vi "Image_Handler.vi"(0 "Camera":T5, 5 "Data":T2={"system"={"info"={"menuSelect"=0, "version"=0, "serial"="Test Sample", "captureActive"=FALSE, "captureBegin"=FALSE, "emptyAndRefill"=FALSE}, "userInfo"={"operatorName"="", "date"=timestamp(2713993200 s since 1904-01-01)}, "camera"={"exposureTime"=0, "aperture"=enum."Item 0", "framerate"=0, "framerateMax"=500, "legacyAttributes"=FALSE}}, "connections"={"arduino"={"connection"="MRJ", "status"=FALSE, "openState"=FALSE, "emptyStart"=0}, "pump"={"connection"="MRJ", "status"=FALSE, "command"="", "dispenseSpeed"=100, "flushSize"=100}, "camera"={"cam1"={"connection"="", "status"=FALSE}, "cam2"={"connection"="", "status"=FALSE}}}, "queue"={"process"={"cam1"=refnum, "cam2"=refnum, "queueSize"=0}, "save"={"cam1"=refnum, "cam2"=refnum, "queueSize"=0}, "overloadThreshold"=0}, "imageProcess"={"cam1"={"preAllocation"={"image"="Station", "originalDisplay"="Station", "originalRgb"="Station", "binary"="Station", "save"="Station", "calibrationFull"=refnum, "calibrationDetect"=refnum}, "calibration"={"pathFull"=path "C:/Users/au540322/Desktop/IHS_Project/images/Debris/Debris_0/Debris_0_2019_06_01-23-32-49-686.PNG", "pathDetect"=path "C:/Users/au540322/Desktop/IHS_Project/images/Debris/Debris_0/Debris_0_2019_06_01-23-32-49-686.PNG", "ROI"={"Left"=0, "Top"=0, "Right"=0, "Bottom"=0, "Rotation"=0.0}}}, "cam2"={"preAllocation"={"image"=refnum, "originalDisplay"=refnum, "originalRgb"=refnum, "binary"=refnum, "save"=refnum, "calibrationFull"=refnum, "calibrationDetect"=refnum}, "calibration"={"pathFull"=path "C:/Users/au540322/Desktop/IHS_Project/images/Debris/Debris_0/Debris_0_2019_06_01-23-32-49-686.PNG", "pathDetect"=path "C:/Users/au540322/Desktop/IHS_Project/images/Debris/Debris_0/Debris_0_2019_06_01-23-32-49-686.PNG", "ROI"={"Left"=0, "Top"=0, "Right"=0, "Bottom"=0, "Rotation"=0.0}}}, "process"={"planeExtract"=refnum, "planeSubtract"=refnum, "cropMask"=refnum}, "detection"={"sampleTimeout"=500, "sizeThreshold"=500, "detectionRegionPct"=0.0}}, "sampleData"={"sampleId"="", "projectId"="", "voucherID"="", "speciesName"="", "collectionDate"=timestamp(2713993200 s since 1904-01-01), "sampleStation"="", "location"="", "lat"=0.0, "lon"=0.0, "determiner"="", "sex"="", "otherNotes"=""}, "Session In"=""} {"sampleData"."collectionDate" format="%<%Y-%m-%d>T"; "imageProcess"."detection"."sizeThreshold" min=1; "imageProcess"."cam2"."calibration"."ROI"."Rotation" format="%.2f"; "imageProcess"."cam2"."calibration"."ROI"."Left" scale=0.0..1024.0; "imageProcess"."cam2"."calibration"."ROI"."Right" scale=0.0..1024.0; "imageProcess"."cam1"."calibration"."ROI"."Rotation" format="%.2f"; "imageProcess"."cam1"."calibration"."ROI"."Left" scale=0.0..1024.0; "imageProcess"."cam1"."calibration"."ROI"."Right" scale=0.0..1024.0; "queue"."overloadThreshold" min=1; "queue"."save"."queueSize" min=1; "queue"."process"."queueSize" min=1; "connections"."pump"."flushSize" min=1; "connections"."pump"."dispenseSpeed" min=1; "system"."camera"."framerateMax" min=1; "system"."userInfo"."date" format="%<%Y-%m-%dT%H:%M:%S+%z>T"; "system"."info"."version" items=["Standard", "XL"]; "system"."info"."menuSelect" items=["Session Data", "Extended Setup", "Buffer", "Camera", "Dispenser", "Stats", "Connections"]}, 9 "Prev. sample":i32, 11 "Timeout in":i32) -> (2 "Detection error":errorcluster, 3 "Object":bool, 4 "Detected object":T1, 6 "Image Out":T1, 8 "Binary":T1, 10 "Sample nr":i32, 15 "Timeout out":i32)   [LabVIEW 2022 SP3]
uses:
  Camera_ID.ctl
  controls/Data.ctl
  <vilib>/userdefined/High Color/IMAQdx.ctl
  <vilib>/vision/Image Controls.llb/IMAQ Image.ctl
panel:
  out "error out 1":errorcluster
  out "error out 2":errorcluster
  in  "error in":errorcluster
  out "error out":errorcluster
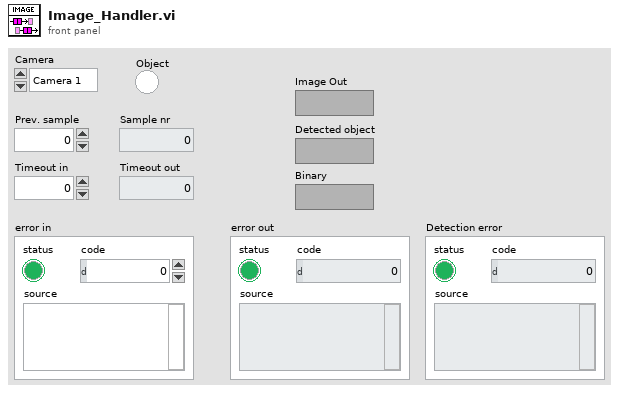
[diagram p1: front panel]
types:
  T1 = typedef "IMAQ Image.ctl" = refnum<image>
  T2 = typedef "Data.ctl" = cluster{"system":cluster{"info":cluster{"menuSelect":u16, "version":u16, "serial":string, "captureActive":bool, "captureBegin":bool, "emptyAndRefill":bool}, "userInfo":cluster{"operatorName":string, "date":timestamp}, "camera":cluster{"exposureTime":i32, "aperture":enum32{"Item 0", "Item 1", "Item 2", "Item 3"}, "framerate":i32, "framerateMax":i32, "legacyAttributes":bool}}, "connections":cluster{"arduino":cluster{"connection":refnum<visa-resource-name>, "status":bool, "openState":bool, "emptyStart":u32}, "pump":cluster{"connection":refnum<visa-resource-name>, "status":bool, "command":string, "dispenseSpeed":i32, "flushSize":i32}, "camera":cluster{"cam1":cluster{"connection":T3, "status":bool}, "cam2":cluster{"connection":T3, "status":bool}}}, "queue":cluster{"process":cluster{"cam1":refnum<queue>, "cam2":refnum<queue>, "queueSize":i32}, "save":cluster{"cam1":refnum<queue>, "cam2":refnum<queue>, "queueSize":i32}, "overloadThreshold":i32}, "imageProcess":cluster{"cam1":cluster{"preAllocation":cluster{"image":T1, "originalDisplay":T1, "originalRgb":T1, "binary":T1, "save":T1, "calibrationFull":T1, "calibrationDetect":T1}, "calibration":cluster{"pathFull":path, "pathDetect":path, "ROI":T4}}, "cam2":cluster{"preAllocation":cluster{"image":T1, "originalDisplay":T1, "originalRgb":T1, "binary":T1, "save":T1, "calibrationFull":T1, "calibrationDetect":T1}, "calibration":cluster{"pathFull":path, "pathDetect":path, "ROI":T4}}, "process":cluster{"planeExtract":T1, "planeSubtract":T1, "cropMask":T1}, "detection":cluster{"sampleTimeout":i32, "sizeThreshold":i32, "detectionRegionPct":dbl}}, "sampleData":cluster{"sampleId":string, "projectId":string, "voucherID":string, "speciesName":string, "collectionDate":timestamp, "sampleStation":string, "location":string, "lat":dbl, "lon":dbl, "determiner":string, "sex":string, "otherNotes":string}, "Session In":T3}
  T3 = typedef "IMAQdx.ctl" = refnum<k21>
  T4 = typedef "IMAQ Rectangle" = cluster{"Left":i32, "Top":i32, "Right":i32, "Bottom":i32, "Rotation":dbl}
  T5 = typedef "Camera_ID.ctl" = enum16{"Camera 1", "Camera 2"}
  T6 = cluster{"Image Pixels (U32)":u32[][], "Detect Movement":bool}
  T7 = cluster{"Global Rectangle":i32[], "Contours":cluster{"ID":enum32{"External", "Internal"}, "Type":u32, "Coordinates":i32[]}[]}
  T8 = cluster{"Timestamp":string, "Image Pixels (U32)":u32[][], "Prev. sample":i32, "Sample Data":dbl[], "ROI descriptor":cluster{"Global Rectangle":i32[], "Contours":cluster{"ID":enum32{"External", "Internal"}, "Type":u32, "Coordinates":i32[]}[]}}
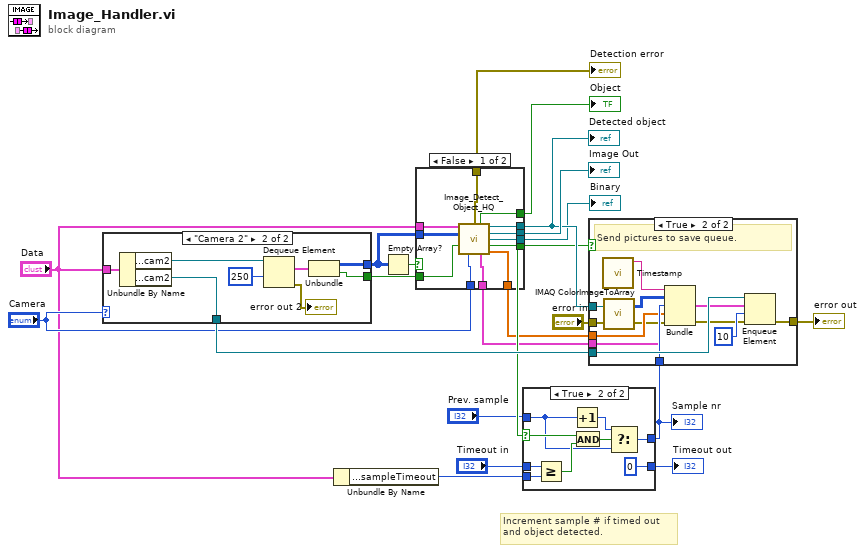
[diagram p0: block diagram]
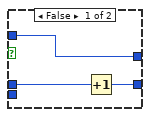
[diagram p2: hidden frame]
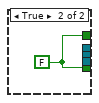
[diagram p4: hidden frame]
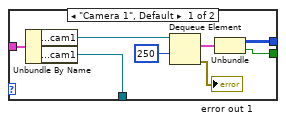
[diagram p5: hidden frame]
diagram:
  # "Increment sample # if timed out \nand object detected."
  n1 = case shown="\"Camera 2\"" "Camera" {
    tunnel: "Data" -> [w29 w37]
    tunnel: [w25 w32] -> w18
    tunnel: [w24 w31] -> w9
    tunnel: [w23 w30] -> w5
    frame "Camera 1", Default {
      n2 = Unbundle By Name(w29) -> ("queue.process.cam1"=w27:refnum<queue>, "queue.save.cam1"=w25:refnum<queue>)
      n3 = Dequeue Element(queue=w27, timeout in ms (-1)=250) -> (element=w22:T6, error out=→"error out 1":errorcluster)  [unwired: 1 in, 2 out]
      n4 = Unbundle(w22) -> ("Image Pixels (U32)"=w24:u32[][], "Detect Movement"=w23:bool)
    }
    frame "Camera 2" {
      n5 = Unbundle By Name(w37) -> ("queue.process.cam2"=w35:refnum<queue>, "queue.save.cam2"=w32:refnum<queue>)
      n6 = Dequeue Element(queue=w35, timeout in ms (-1)=250) -> (element=w34:T6, error out=→"error out 2":errorcluster)  [unwired: 1 in, 2 out]
      n7 = Unbundle(w34) -> ("Image Pixels (U32)"=w31:u32[][], "Detect Movement"=w30:bool)
    }
  }
  n8 = Unbundle By Name("Data") -> ("imageProcess.detection.sampleTimeout"=w11:i32)
  n9 = Empty Array?(array=w9) -> (empty?=w21:bool)
  n10 = case shown="False" w21 {
    tunnel: [w49 _] -> w19
    tunnel: [w41 w50] -> w14
    tunnel: "Data" -> [w48 _]
    tunnel: "Camera" -> [w47 _]
    tunnel: [w46 _] -> w20
    tunnel: w9 -> [w45 _]
    tunnel: [w44 w50] -> w6
    tunnel: w5 -> [w43 _]
    tunnel: [w42 _] -> w4
    tunnel: [w40 _] -> w3
    tunnel: [w39 _] -> w2
    tunnel: [w38 _] -> w1
    frame False {
      n11 = call "Image_Detect_Object_HQ.vi"("Data"=w48, "Image Pixels (U32)"=w45, "Detect Crop"=w43, "Camera"=w47) -> ("error out"=w38:errorcluster, "Obj Size"=w44:bool, "Detected object"=w49:T1, "Image Out"=w46:T1, "Binary"=w40:T1, "Object Accept"=w41:bool, "ROI descriptor"=w39:T7, "Sample Data"=w42:dbl[])  [unwired: 4 in]
    }
    frame True {
      w50 = FALSE ("Object detected")
    }
  }
  "Detected object" <- w19
  "Image Out" <- w20
  "Binary" <- w3
  "Object" <- w6
  "Detection error" <- w1
  n12 = case shown="True" w14 {
    selector: w14 -> [_ w62]
    tunnel: w11 -> [_ w61]
    tunnel: [w53 0] -> w12
    tunnel: [w52 w56] -> w10
    tunnel: "Prev. sample" -> [w52 w55]
    tunnel: "Timeout in" -> [w51 w54]
    frame False {
      n13 = Increment(x=w51) -> (x+1=w53:i32)
    }
    frame True {
      n14 = Greater Or Equal?(x=w54, y=w61) -> (x >= y?=w60:bool)
      n15 = Increment(x=w55) -> (x+1=w57:i32)
      n16 = And(x=w62, y=w60) -> (x .and. y?=w58:bool)
      n17 = Select(t=w57, s=w58, f=w55) -> (s? t:f=w56:i32)
    }
  }
  "Sample nr" <- w10
  "Timeout out" <- w12
  n18 = case shown="True" w14 {
    tunnel: w19 -> [_ w69]
    tunnel: w18 -> [_ w75]
    tunnel: "error in" -> [w63 w68]
    tunnel: [w63 w74] -> w15
    tunnel: w10 -> [_ w72]
    tunnel: w4 -> [_ w70]
    tunnel: w2 -> [_ w64]
    frame False {
      # "No object within criteria."
    }
    frame True {
      # "Send pictures to save queue."
      n19 = call "Timestamp.vi"() -> ("Timestamp"=w73:string)  [unwired: 11 in]
      n20 = call "IMAQ ColorImageToArray"("Image"=w69, "error in (no error)"=w68) -> ("Image Pixels (U32)"=w66:u32[][], "error out"=w67:errorcluster)  [unwired: 2 in, 1 out]
      n21 = Bundle("Timestamp"=w73, "Image Pixels (U32)"=w66, "Prev. sample"=w72, "Sample Data"=w70, "ROI descriptor"=w64) -> (w65:T8)  [unwired: 1 in]
      n22 = Enqueue Element(queue=w75, element=w65, timeout in ms (-1)=10, error in (no error)=w67) -> (error out=w74:errorcluster)  [unwired: 2 out]
    }
  }
  "error out" <- w15
